vi "VisionMain.vi"(6 "Generated Distance Array":dbl[][](array[numeric]), 8 "Y Center":dbl, 9 "X Center":dbl, 10 "Original Plots":T1(array[cluster]), 11 "Plots Captured":T1(array[cluster])) -> (1 "alpha":dbl, 2 "dy":dbl, 3 "dx":dbl)   [LabVIEW 2012]
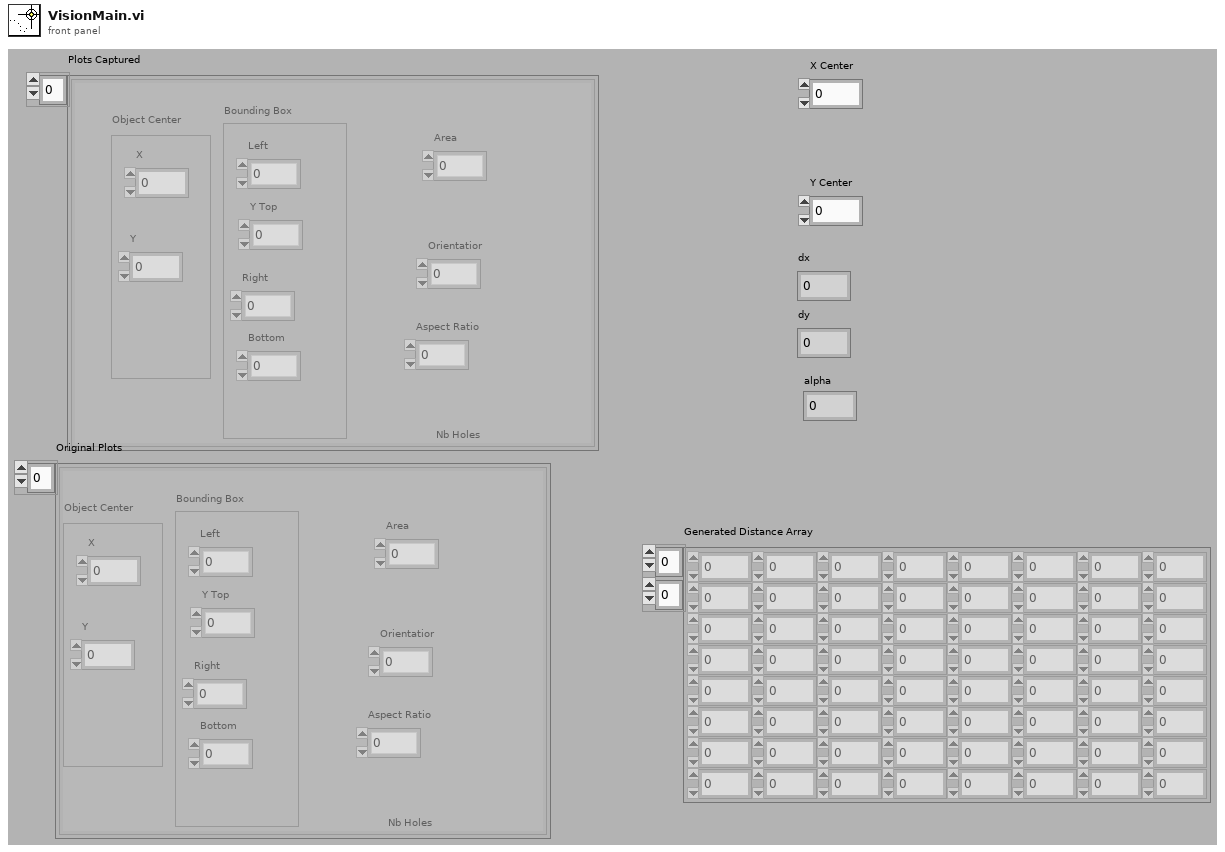
[diagram p1: front panel]
types:
  T1 = cluster{"Object Center":cluster{"X":dbl, "Y":dbl}, "Bounding Box":cluster{"Left":dbl, "Right":dbl, "Bottom":dbl, "Y Top":dbl}, "Area":dbl, "Orientatior":dbl, "Aspect Ratio":dbl, "Nb Holes":dbl}[]
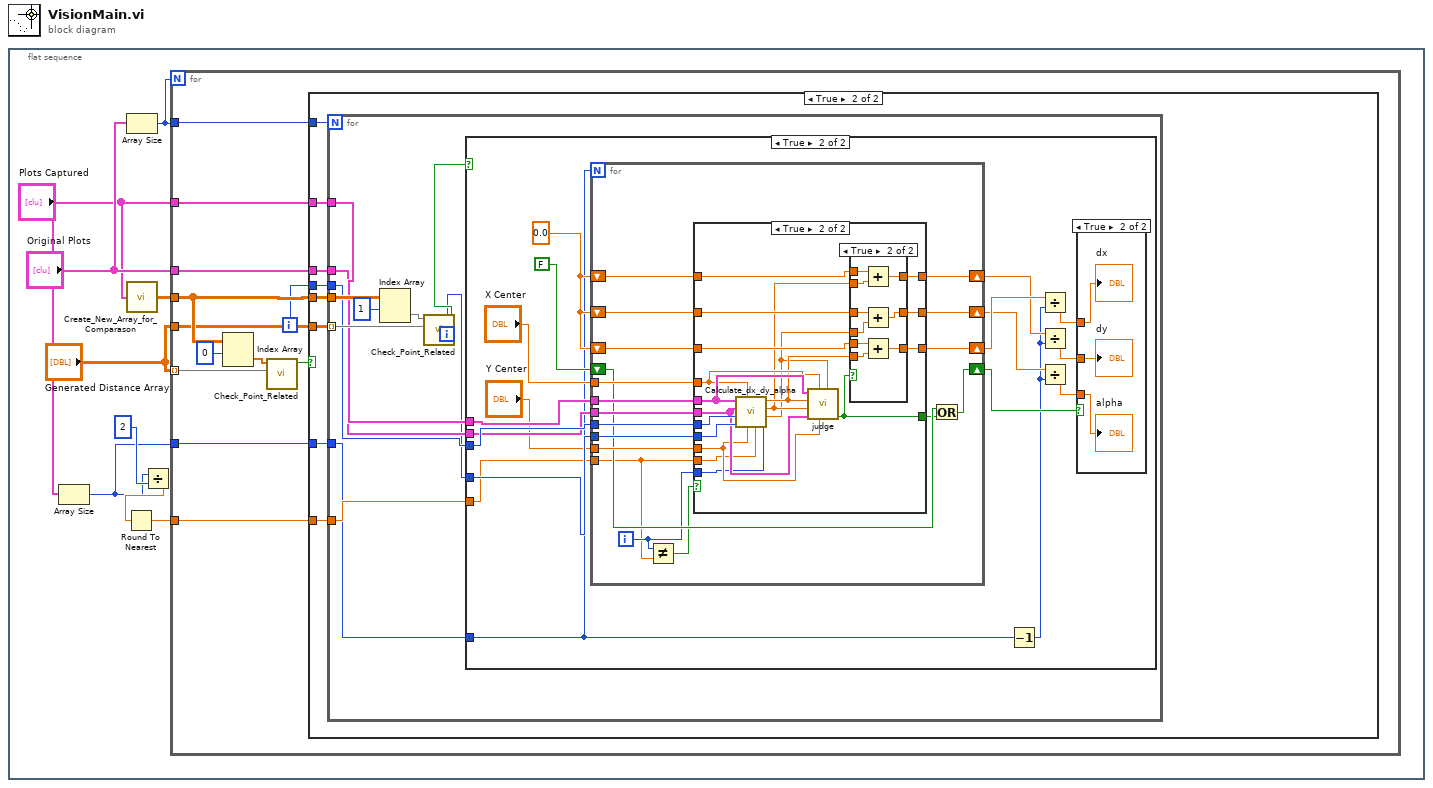
[diagram p0: block diagram]
diagram:
  n1 = flat-sequence {
    frame #0 {
      n2 = Array Size(array="Plots Captured") -> (size(s)=w1:i32)
      n3 = Array Size(array="Original Plots") -> (size(s)=w7:i32)
      n4 = call "Create_New_Array_for_Comparason.vi"("Captured Plots"="Plots Captured") -> ("Generated Distance Array"=w9:dbl[][])
      n5 = Divide(x=w1, y=2) -> (x/y=w3:dbl)
      n6 = Round To Nearest(number=w3) -> (nearest integer value=w2:dbl)
      n7 = for {
        N: w7 -> [_]
        tunnel: w9 -> [w18]
        tunnel: "Generated Distance Array" -> [w17] mode=indexing
        tunnel: "Generated Distance Array" -> [w16]
        tunnel: "Plots Captured" -> [w15]
        tunnel: "Original Plots" -> [w14]
        tunnel: w7 -> [w12]
        tunnel: w2 -> [w11]
        tunnel: w1 -> [w10]
        i -> [w13]
        n8 = Index Array(array=w18, index (row)=0) -> (element=w20:dbl[])  [unwired: 1 in]
        n9 = call "Check_Point_Related.vi"("Original Plots"=w17, "Captured Plots"=w20) -> ("result"=w19:bool)  [unwired: 9 in]
        n10 = case shown="True" w19 {
          tunnel: w18 -> [_ w29]
          tunnel: w16 -> [_ w28]
          tunnel: w15 -> [_ w27]
          tunnel: w14 -> [_ w26]
          tunnel: w13 -> [_ w25]
          tunnel: w12 -> [_ w24]
          tunnel: w11 -> [_ w23]
          tunnel: w10 -> [_ w22]
          frame False {
          }
          frame True {
            n11 = for {
              N: w24 -> [_]
              tunnel: w29 -> [w40]
              tunnel: w28 -> [w36] mode=indexing
              tunnel: w27 -> [w35]
              tunnel: w26 -> [w34]
              tunnel: w25 -> [w33]
              tunnel: w23 -> [w31]
              tunnel: w22 -> [w30]
              i -> [w32]
              n12 = Index Array(array=w40, index (row)=1) -> (element=w38:dbl[])  [unwired: 1 in]
              n13 = call "Check_Point_Related.vi"("Original Plots"=w36, "Captured Plots"=w38) -> ("result"=w37:bool)  [unwired: 9 in]
              n14 = case shown="True" w37 {
                tunnel: w35 -> [_ w56]
                tunnel: w34 -> [_ w55]
                tunnel: w33 -> [_ w58]
                tunnel: w32 -> [_ w57]
                tunnel: w31 -> [_ w52]
                tunnel: w30 -> [_ w42]
                frame False {
                }
                frame True {
                  w51 = 0.0
                  n15 = for {
                    N: w42 -> [_]
                    tunnel: w58 -> [w76]
                    tunnel: w57 -> [w75]
                    tunnel: w56 -> [w74]
                    tunnel: w55 -> [w73]
                    tunnel: "X Center" -> [w72]
                    tunnel: "Y Center" -> [w71]
                    tunnel: w52 -> [w60]
                    shift-right: [w67] -> w48
                    shift-left: w51 -> [w69]
                    shift-right: [w65] -> w46
                    shift-left: w51 -> [w68]
                    shift-right: [w66] -> w50
                    shift-left: w51 -> [w70]
                    shift-right: [w62] -> w43
                    shift-left: FALSE -> [w64]
                    i -> [w61]
                    n16 = Not Equal?(x=w61, y=w60) -> (x != y?=w59:bool)
                    n17 = case shown="True" w59 {
                      selector: w59 -> [w77 _]
                      tunnel: w76 -> [_ w98]
                      tunnel: w75 -> [_ w97]
                      tunnel: w74 -> [_ w96]
                      tunnel: w73 -> [_ w95]
                      tunnel: w72 -> [_ w94]
                      tunnel: w71 -> [_ w93]
                      tunnel: w70 -> [w80 w92]
                      tunnel: w69 -> [w79 w91]
                      tunnel: w68 -> [w78 w90]
                      tunnel: [w79 w86] -> w67
                      tunnel: [w80 w85] -> w66
                      tunnel: [w78 w84] -> w65
                      tunnel: [w77 w83] -> w63
                      tunnel: w61 -> [_ w82]
                      tunnel: w60 -> [_ w81]
                      frame False {
                      }
                      frame True {
                        n18 = call "Calculate_dx_dy_alpha.vi"("index 2"=w82, "index 1"=w81, "c_y"=w93, "c_x"=w94, "Corresponding Point #2"=w97, "Corresponding Point #1"=w98, "Original Plots"=w95, "Captured Plots"=w96) -> ("alpha"=w87:dbl, "dy"=w88:dbl, "dx"=w89:dbl)  [unwired: 1 in]
                        n19 = call "judge.vi"("alpha"=w87, "c_y"=w93, "c_x"=w94, "Original Plots"=w95, "dy"=w88, "dx"=w89, "Captured Plots"=w96) -> ("result"=w83:bool)  [unwired: 4 in]
                        n20 = case shown="True" w83 {
                          tunnel: w92 -> [w101 w110]
                          tunnel: w91 -> [w100 w109]
                          tunnel: w90 -> [w99 w108]
                          tunnel: w89 -> [_ w107]
                          tunnel: w88 -> [_ w106]
                          tunnel: w87 -> [_ w105]
                          tunnel: [w101 w104] -> w85
                          tunnel: [w100 w103] -> w86
                          tunnel: [w99 w102] -> w84
                          frame False {
                          }
                          frame True {
                            n21 = Add(x=w109, y=w106) -> (x+y=w103:dbl)
                            n22 = Add(x=w108, y=w105) -> (x+y=w102:dbl)
                            n23 = Add(x=w110, y=w107) -> (x+y=w104:dbl)
                          }
                        }
                      }
                    }
                    n24 = Or(x=w64, y=w63) -> (x .or. y?=w62:bool)
                  }
                  n25 = Decrement(x=w42) -> (x-1=w41:i32)
                  n26 = Divide(x=w50, y=w41) -> (x/y=w49:dbl)
                  n27 = Divide(x=w48, y=w41) -> (x/y=w47:dbl)
                  n28 = Divide(x=w46, y=w41) -> (x/y=w45:dbl)
                  n29 = case shown="True" w43 {
                    tunnel: w49 -> [_ w113]
                    tunnel: w47 -> [_ w112]
                    tunnel: w45 -> [_ w111]
                    frame False {
                    }
                    frame True {
                      "dx" <- w113
                      "dy" <- w112
                      "alpha" <- w111
                    }
                  }
                }
              }
            }
          }
        }
      }
    }
  }
